vi "写入数据.vi"(6 "tdms文件":refnum<k34>, 7 "组名称输入（无标题）":string, 8 "错误输入（无错误）":errorcluster, 11 "测试数据":dbl[][](array[numeric])) -> (0 "错误输出":errorcluster, 4 "tdms文件输出":refnum<k34>, 5 "组名称输出":string)   [LabVIEW 2021]
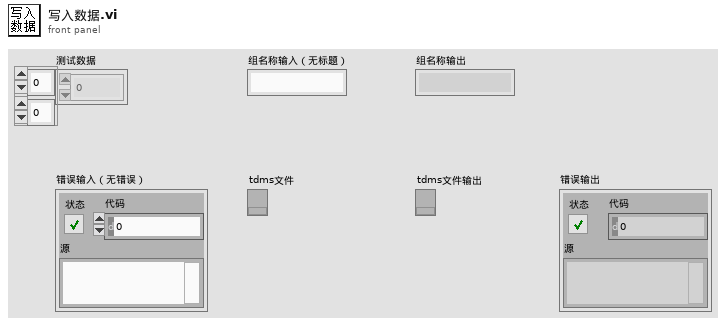
[diagram p1: front panel]
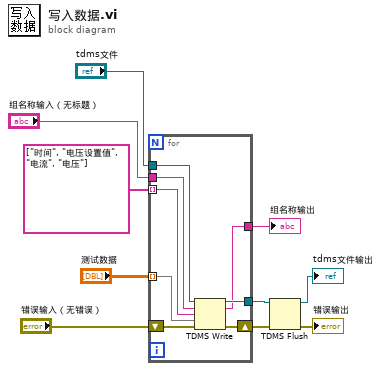
[diagram p0: block diagram]
diagram:
  n1 = for {
    tunnel: "tdms文件" -> [w18]
    tunnel: string[] ["时间", "电压设置值", "电流", "电压"] -> [w12] mode=indexing
    shift-right: [w16] -> w7
    shift-left: "错误输入（无错误）" -> [w17]
    tunnel: [w15] -> w6
    tunnel: [w14] -> w5
    tunnel: "测试数据" -> [w13] mode=indexing
    tunnel: "组名称输入（无标题）" -> [w11]
    n2 = TDMS Write(0:w18, 5:w11, 7:w12, 9:w13, 11:w17) -> (4:w15:refnum<k34>, 6:w14:string, 15:w16:errorcluster)  [unwired: 1 in, 1 out]
  }
  "组名称输出" <- w5
  n3 = TDMS Flush(4:w7, 7:w6) -> (0:→"错误输出":errorcluster, 3:→"tdms文件输出":refnum<k34>)
